vi "unbuild waveform array_4.vi"(10 "Array":waveform(dbl)[](array[waveform])) -> (0 "4":dbl, 1 "3":dbl, 2 "2":dbl, 3 "1":dbl, 4 "débits":cluster{dbl, dbl, dbl, dbl})   [LabVIEW 2014]
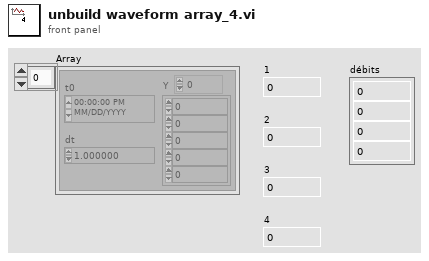
[diagram p1: front panel]
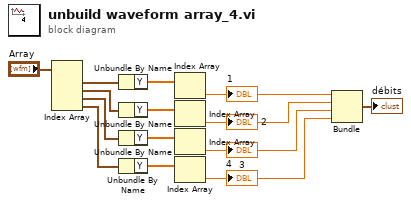
[diagram p0: block diagram]
diagram:
  n1 = Index Array(array="Array") -> (element #1=w7:waveform(dbl), element #2=w8:waveform(dbl), element #3=w9:waveform(dbl), element #4=w10:waveform(dbl))  [unwired: 4 in]
  n2 = Unbundle By Name(w7) -> ("Y"=w11:dbl[])
  n3 = Unbundle By Name(w8) -> ("Y"=w12:dbl[])
  n4 = Unbundle By Name(w9) -> ("Y"=w13:dbl[])
  n5 = Unbundle By Name(w10) -> ("Y"=w14:dbl[])
  n6 = Index Array(array=w11) -> (element=w5:dbl)  [unwired: 1 in]
  "1" <- w5
  n7 = Index Array(array=w12) -> (element=w4:dbl)  [unwired: 1 in]
  "2" <- w4
  n8 = Index Array(array=w13) -> (element=w3:dbl)  [unwired: 1 in]
  "3" <- w3
  n9 = Index Array(array=w14) -> (element=w2:dbl)  [unwired: 1 in]
  "4" <- w2
  n10 = Bundle(w5, w4, w3, w2) -> (→"débits":cluster{dbl, dbl, dbl, dbl})  [unwired: 1 in]
